vi "GLOBAL -MAIN.vi"() -> ()   [LabVIEW 2011]
panel:
  out "EXIT":bool
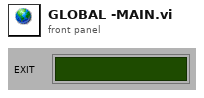
[diagram p1: front panel]
diagram:
